vi "ActuatorOutput.vi"(8 "error in (no error)":errorcluster, 11 "Cluster in":T1) -> (0 "error out":errorcluster, 3 "Cluster":T1)   [LabVIEW 2018]
uses:
  Type_Def/Type_Def Actuator Controls.ctl
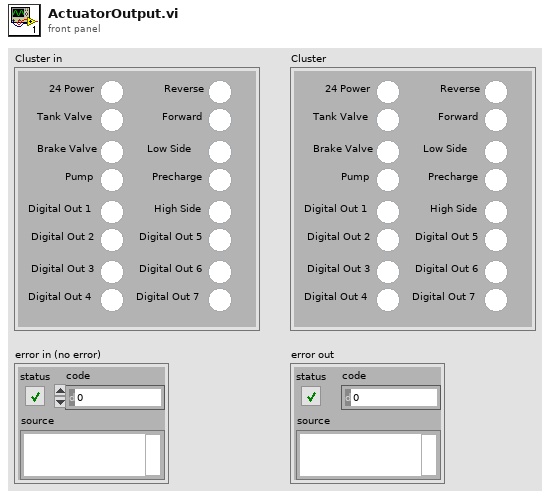
[diagram p1: front panel]
types:
  T1 = typedef "Type_Def Actuator Controls.ctl" = cluster{"Reverse ":bool, "Forward":bool, "Low Side":bool, "Precharge":bool, "High Side":bool, "Digital Out 5":bool, "Digital Out 6":bool, "Digital Out 7 ":bool, "24 Power":bool, "Tank Valve ":bool, "Brake Valve":bool, "Pump":bool, "Digital Out 1 ":bool, "Digital Out 2":bool, "Digital Out 3":bool, "Digital Out 4 ":bool}
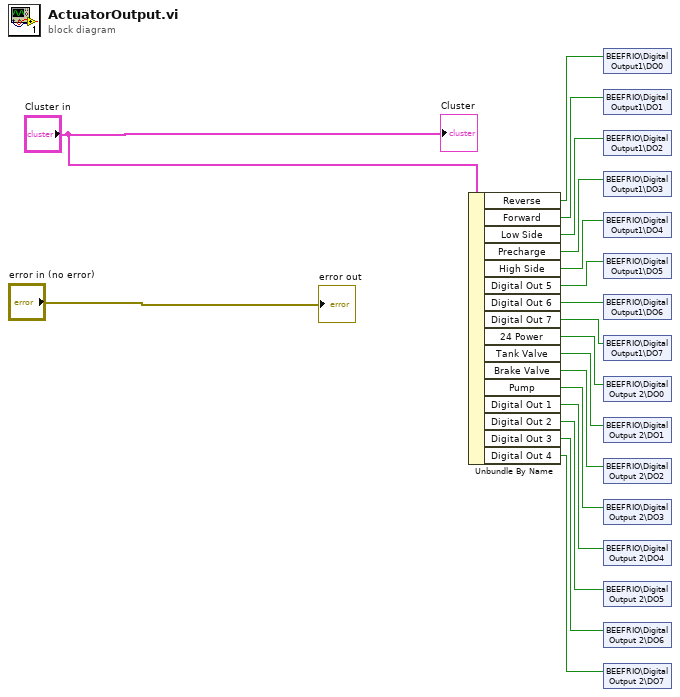
[diagram p0: block diagram]
diagram:
  n1 = Unbundle By Name("Cluster in") -> ("Reverse"=w16:bool, "Forward"=w15:bool, "Low Side"=w14:bool, "Precharge"=w13:bool, "High Side"=w12:bool, "Digital Out 5"=w11:bool, "Digital Out 6"=w10:bool, "Digital Out 7"=w9:bool, "24 Power"=w8:bool, "Tank Valve"=w7:bool, "Brake Valve"=w6:bool, "Pump"=w5:bool, "Digital Out 1"=w4:bool, "Digital Out 2"=w3:bool, "Digital Out 3"=w2:bool, "Digital Out 4"=w1:bool)
  n2 = shared-variable "BEEFRIO\\Digital Output1\\DO0"(w16) -> ()  [unwired: 1 in, 1 out]
  n3 = shared-variable "BEEFRIO\\Digital Output1\\DO1"(w15) -> ()  [unwired: 1 in, 1 out]
  n4 = shared-variable "BEEFRIO\\Digital Output1\\DO2"(w14) -> ()  [unwired: 1 in, 1 out]
  n5 = shared-variable "BEEFRIO\\Digital Output1\\DO3"(w13) -> ()  [unwired: 1 in, 1 out]
  n6 = shared-variable "BEEFRIO\\Digital Output1\\DO4"(w12) -> ()  [unwired: 1 in, 1 out]
  n7 = shared-variable "BEEFRIO\\Digital Output1\\DO5"(w11) -> ()  [unwired: 1 in, 1 out]
  n8 = shared-variable "BEEFRIO\\Digital Output1\\DO6"(w10) -> ()  [unwired: 1 in, 1 out]
  n9 = shared-variable "BEEFRIO\\Digital Output1\\DO7"(w9) -> ()  [unwired: 1 in, 1 out]
  n10 = shared-variable "BEEFRIO\\Digital Output 2\\DO0"(w8) -> ()  [unwired: 1 in, 1 out]
  n11 = shared-variable "BEEFRIO\\Digital Output 2\\DO1"(w7) -> ()  [unwired: 1 in, 1 out]
  n12 = shared-variable "BEEFRIO\\Digital Output 2\\DO2"(w6) -> ()  [unwired: 1 in, 1 out]
  n13 = shared-variable "BEEFRIO\\Digital Output 2\\DO3"(w5) -> ()  [unwired: 1 in, 1 out]
  n14 = shared-variable "BEEFRIO\\Digital Output 2\\DO4"(w4) -> ()  [unwired: 1 in, 1 out]
  n15 = shared-variable "BEEFRIO\\Digital Output 2\\DO5"(w3) -> ()  [unwired: 1 in, 1 out]
  n16 = shared-variable "BEEFRIO\\Digital Output 2\\DO6"(w2) -> ()  [unwired: 1 in, 1 out]
  n17 = shared-variable "BEEFRIO\\Digital Output 2\\DO7"(w1) -> ()  [unwired: 1 in, 1 out]
  "error out" <- "error in (no error)"
  "Cluster" <- "Cluster in"
